vi "ErrorLog_LogError.vi"(7 "Owner (\"Error\")":string="Error", 8 "error in (no error)":errorcluster, 9 "Context (\"Error\")":string="Error", 10 "Error To Log":errorcluster, 11 "reference in":refnum<class "ErrorLog.lvclass">) -> (0 "error out":errorcluster, 1 "Error String":string, 2 "Cleaned Error":errorcluster, 3 "reference out":refnum<class "ErrorLog.lvclass">, 4 "Error was Logged":bool)   [LabVIEW 2014, in "ErrorLog.lvclass"]
uses:
  ErrorLog.lvclass
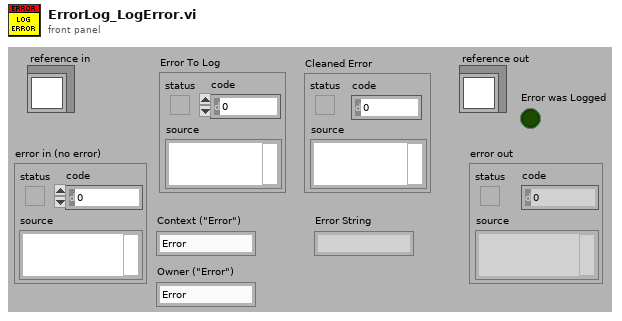
[diagram p1: front panel]
types:
  T1 = typedef "ErrorLog.lvclass/ObjectAttributes.ctl" = cluster{"ErrorFile":path, "Supress Consecutive Duplicates":bool, "Errors":string, "Quit":bool, "Errors since last call":string, "Last Recorded Error":string, "ErrorPath":path, "PossiblePaths":path[], "BaseFileName":string, "Max Log Files":i32, "ErrorFile Index":i32, "Max File Size":i64}
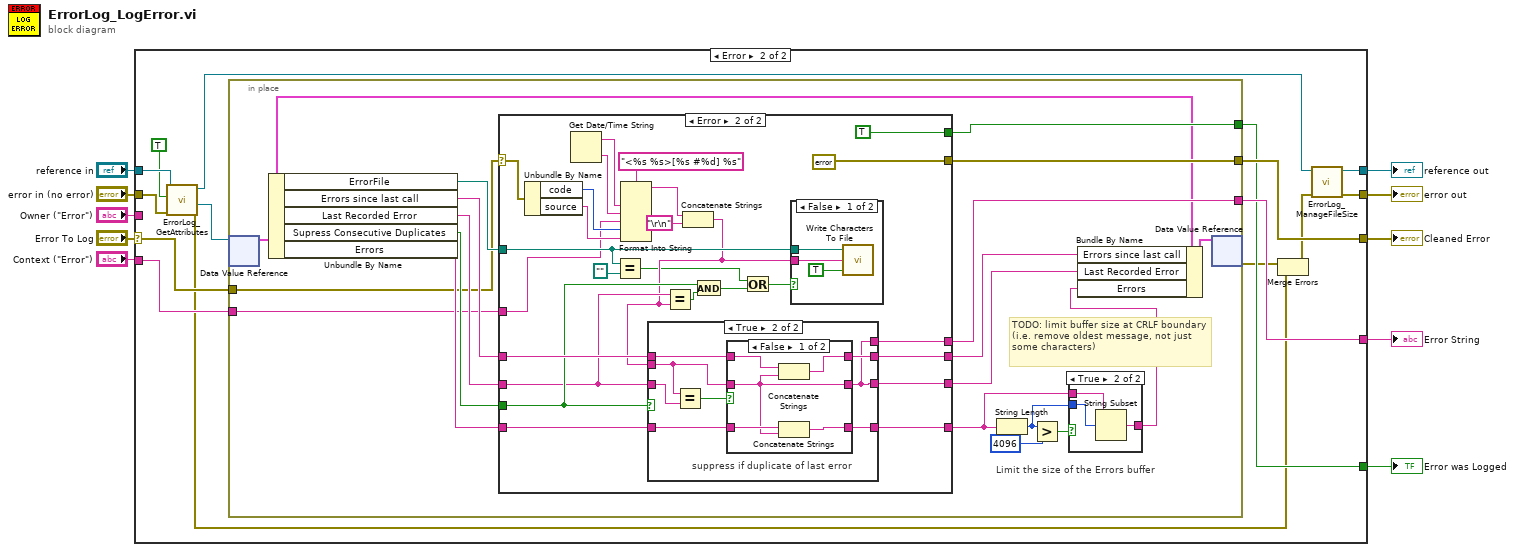
[diagram p0: block diagram]
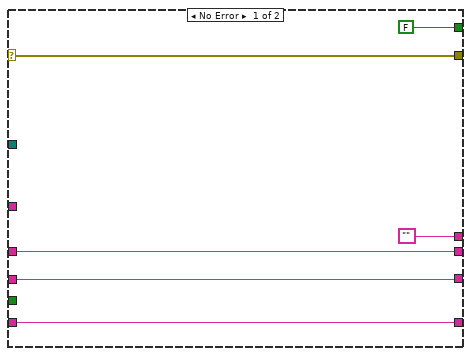
[diagram p4: hidden frame]
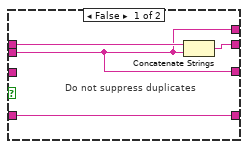
[diagram p6: hidden frame]
diagram:
  n1 = case shown="Error" "Error To Log" {
    selector: "Error To Log" -> [w12 w20]
    tunnel: [w12 w16] -> w10
    tunnel: [w11 w13] -> w8
    tunnel: "reference in" -> [w11 w27]
    tunnel: [_ w22] -> w7
    tunnel: [_ w24] -> w6
    tunnel: "error in (no error)" -> [_ w26]
    tunnel: "Context (\"Error\")" -> [_ w19]
    tunnel: [_ w23] -> w2
    tunnel: "Owner (\"Error\")" -> [_ _]
    frame No Error {
    }
    frame Error {
      n2 = call "ErrorLog_GetAttributes.vi"("error in (no error)"=w26, "OnlyGetDvrReference(False)"=TRUE, "reference in"=w27) -> ("error out"=w17:errorcluster, "DataRef"=w21:refnum<data-value>, "reference out"=w14:refnum<class "ErrorLog.lvclass">)  [unwired: 5 in, 1 out]
      n3 = in-place {
        in-place-border: [w34] -> w24
        in-place-border: [w33] -> w23
        in-place-border: [w32] -> w22
        in-place-border: w20 -> [w29]
        in-place-border: w19 -> [w28]
        # "TODO: limit buffer size at CRLF boundary (i.e. remove oldest message, not just some characters)"
        # "Limit the size of the Errors buffer"
        n4 = in-place-dvr #1(w21) -> (w31:T1)  [unwired: 1 out]
        n5 = Unbundle By Name(w31) -> ("ErrorFile"=w46:path, "Errors since last call"=w45:string, "Last Recorded Error"=w44:string, "Supress Consecutive Duplicates"=w43:bool, "Errors"=w40:string)
        n6 = case shown="Error" w29 {
          selector: w29 -> [w56 w81]
          tunnel: [w56 errorcluster {"status"=FALSE, "code"=0, "source"=""} ("error out")] -> w34
          tunnel: w46 -> [_ w68]
          tunnel: w45 -> [w55 w73]
          tunnel: [w55 w72] -> w41
          tunnel: w44 -> [w54 w65]
          tunnel: w43 -> [_ w66]
          tunnel: [w54 w71] -> w42
          tunnel: ["" w70] -> w33
          tunnel: [FALSE TRUE] -> w32
          tunnel: w40 -> [w51 w59]
          tunnel: [w51 w58] -> w36
          tunnel: w28 -> [_ w57]
          frame No Error {
          }
          frame Error {
            n7 = Unbundle By Name(w81) -> ("code"=w76:i32, "source"=w77:string)
            n8 = Get Date/Time String() -> (date string=w74:string, time string=w75:string)  [unwired: 3 in]
            n9 = Equal?(x=w68, y=path "") -> (x = y?=w62:bool)
            n10 = Format Into String(format string="<%s %s>[%s #%d] %s", w74, w75, w57, w76, w77) -> (resulting string=w78:string)  [unwired: 2 in, 1 out]
            n11 = Concatenate Strings(w78, "\r\n") -> (w64:string)
            n12 = case shown="True" w66 {
              tunnel: w73 -> [w89 w95]
              tunnel: w64 -> [w87 w93]
              tunnel: [w88 w94] -> w72
              tunnel: w65 -> [_ w96]
              tunnel: [w87 w92] -> w71
              tunnel: [w87 w92] -> w70
              tunnel: w59 -> [w86 w91]
              tunnel: [w86 w90] -> w58
              frame False {
                # "Do not suppress duplicates"
                n13 = Concatenate Strings(w89, w87) -> (w88:string)
              }
              frame True {
                # "suppress if duplicate of last error"
                n14 = Equal?(x=w93, y=w96) -> (x = y?=w97:bool)
                n15 = case shown="False" w97 {
                  tunnel: w93 -> [w99 w104]
                  tunnel: w95 -> [w102 w105]
                  tunnel: [w101 w105] -> w94
                  tunnel: [w99 w104] -> w92
                  tunnel: w91 -> [w100 w103]
                  tunnel: [w98 w103] -> w90
                  frame False {
                    n16 = Concatenate Strings(w102, w99) -> (w101:string)
                    n17 = Concatenate Strings(w100, w99) -> (w98:string)
                  }
                  frame True {
                    # "do not record again"
                  }
                }
              }
            }
            n18 = Equal?(x=w65, y=w64) -> (x = y?=w67:bool)
            n19 = And(x=w66, y=w67) -> (x .and. y?=w63:bool)
            n20 = Or(x=w62, y=w63) -> (x .or. y?=w61:bool)
            n21 = case shown="False" w61 {
              tunnel: w64 -> [w84 _]
              tunnel: w68 -> [w83 _]
              frame False {
                n22 = call <vilib>:"Write Characters To File.vi"("append to file? (new file:F)"=TRUE, "character string"=w84, "file path (dialog if empty)"=w83) -> ()  [unwired: 2 in, 1 out]
              }
              frame True {
                # "Object may already be destroyed"
                # "No File or suppressed"
              }
            }
          }
        }
        n23 = String Length(string=w36) -> (length=w37:i32)
        n24 = Greater?(x=w37, y=4096) -> (0:w38:bool)
        n25 = case shown="True" w38 {
          tunnel: w37 -> [_ w50]
          tunnel: w36 -> [w47 w49]
          tunnel: [w47 w48] -> w35
          frame False {
          }
          frame True {
            n26 = String Subset(string=w49, offset (0)=w50) -> (substring=w48:string)  [unwired: 1 in]
          }
        }
        n27 = Bundle By Name(cluster=w31, "Errors since last call"=w41, "Last Recorded Error"=w42, "Errors"=w35) -> (w30:T1)
        n28 = in-place-dvr #1(w30) -> (w18:errorcluster)  [unwired: 1 out]
      }
      n29 = Merge Errors(w18, w17) -> (w15:errorcluster)
      n30 = call-dynamic "ErrorLog_ManageFileSize.vi"("error in (no error)"=w15, "reference in"=w14) -> ("error out"=w16:errorcluster, "reference out"=w13:refnum<class "ErrorLog.lvclass">)  [unwired: 8 in]
    }
  }
  "error out" <- w10
  "reference out" <- w8
  "Cleaned Error" <- w6
  "Error was Logged" <- w7
  "Error String" <- w2
